vi "System Config_SubVIs-某型振动实验台测试系统.vi"(8 "Error In":errorcluster) -> (0 "Error Out":errorcluster, 1 "Cancle":bool, 3 "Task Info":T1={"Accele Task"=[], "Simulate"=FALSE, "采样率"={"AISampleRate"=10123, "CouplingType"=10000, "Butter"=1000}, "Trig"={"PreTrigCNT"=0, "TriggerMode"=enum."中间触发", "TriggerSource"=enum."软件触发", "ATRTriggerChannel"=enum."通道0", "TriggerDir"=enum."下降沿触发", "TrigLevelVolt"=0.0, "bAvailableTrig"=FALSE}, "clock"={"EN"=FALSE, "clocksource"=enum."内部时钟", "outclocksource"=enum."Trig0"}, "delay(S)"=0.0} {"采样率"."CouplingType" items=["直流耦合", "交流耦合"]})   [LabVIEW 2011]
uses:
  Ctrls/Task Info.ctl
  Ctrls/Sample Information.ctl
  Ctrls/Trig.ctl
  Ctrls/clock.ctl
  Ctrls/task.ctl
  Ctrls/DATA info.ctl
panel:
  in  "取消":bool
  in  "确认":bool
  in  "Tab Control":enum32{"通道设置", "硬件设置"}(tab)
  in  "Scrollbar":i32(c297)
  in  "Accele":T2[](array[typedef])=[{"Enable"=FALSE, "Name"="", "range"=enum."±1V", "SensValue"=0.0, "PhysicalName"="", "off"=0.0, "Sensunits"=""}, {"Enable"=FALSE, "Name"="", "range"=enum."±1V", "SensValue"=0.0, "PhysicalName"="", "off"=0.0, "Sensunits"=""}, {"Enable"=FALSE, "Name"="", "range"=enum."±1V", "SensValue"=0.0, "PhysicalName"="", "off"=0.0, "Sensunits"=""}, {"Enable"=FALSE, "Name"="", "range"=enum."±1V", "SensValue"=0.0, "PhysicalName"="", "off"=0.0, "Sensunits"=""}]
  in  "All":bool caption="选择全部"
  in  "triglevelvolt":dbl caption="触发值(Mpa)"
  in  "数据保存时间(S)":dbl
  in  "Trig.ctlclock":T5
  in  "SampleInfo":T3={"AISampleRate"=10123, "CouplingType"=10000, "Butter"=1000} {"CouplingType" items=["直流耦合", "交流耦合"]; "AISampleRate" format="%#_6f"}
  in  "PreTrigCNT":i32 caption="预触发数"
  in  "TriggerMode":enum16{"中间触发", "后触发", "预触发", "硬件延时触发"}(ring) caption="触发模式"
  in  "TriggerSource":enum16{"软件触发", "DTR信号源", "ATR信号源", "Triger信号触发"}(ring) caption="触发源"
  in  "ATRTriggerChannel":enum16{"通道0", "通道1", "通道2", "通道3"}(ring) caption="触发通道"
  in  "TriggerDir":enum16{"下降沿触发", "上升沿触发", "上下边没均触发"}(ring) caption="触发方向"
  in  "bAvailableTrig":bool caption="触发事件提前有效么？"
  # "增益"
  # "使用"
  # "物理通道"
  # "通道名称"
  # "灵敏度"
  # "偏差"
  # "单位"
  # "采样"
  # "触发"
  # "时钟"
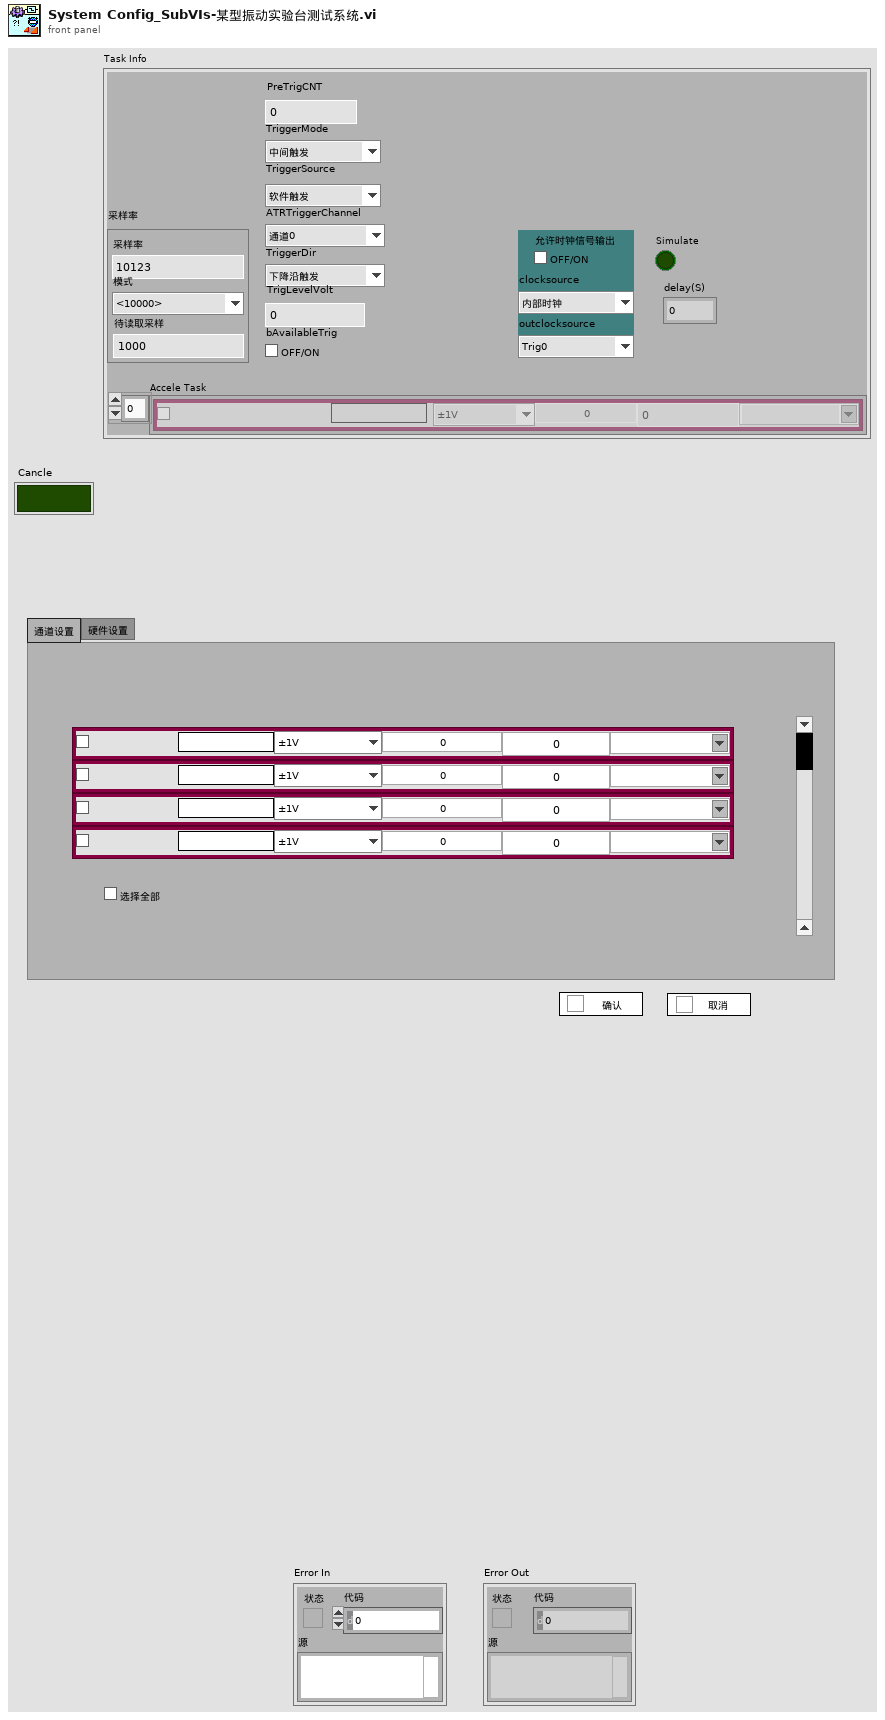
[diagram p1: front panel]
types:
  T1 = typedef "Task Info.ctl" = cluster{"Accele Task":T2[], "Simulate":bool, "采样率":T3, "Trig":T4, "clock":T5, "delay(S)":dbl}
  T2 = typedef "Acceleration Channel Config_Ctrls-某型振动实验台测试系统.ctl" = cluster{"Enable":bool, "Name":string, "range":enum16{"±1V", "±5V"}, "SensValue":dbl, "PhysicalName":string, "off":dbl, "Sensunits":string}
  T3 = typedef "Sample Information.ctl" = cluster{"AISampleRate":i32, "CouplingType":i32, "Butter":i32}
  T4 = typedef "Trig.ctl" = cluster{"PreTrigCNT":i32, "TriggerMode":enum16{"中间触发", "后触发", "预触发", "硬件延时触发"}, "TriggerSource":enum16{"软件触发", "DTR信号源", "ATR信号源", "Triger信号触发"}, "ATRTriggerChannel":enum16{"通道0", "通道1", "通道2", "通道3"}, "TriggerDir":enum16{"下降沿触发", "上升沿触发", "上下边没均触发"}, "TrigLevelVolt":sgl, "bAvailableTrig":bool}
  T5 = typedef "clock.ctl" = cluster{"EN":bool, "clocksource":enum16{"内部时钟", "外部时钟"}, "outclocksource":enum16{"Trig0", "Trig1", "Trig2", "Trig3", "Trig4", "Trig5", "Trig6", "Trig7", "PXI_STAR"}}
  T6 = typedef "Enum Config_Ctrls-某型振动实验台测试系统.ctl" = enum16{"Initialize", "No Action", "Save Config File", "Error Handle", "Exit"}
  T7 = typedef "task.ctl" = cluster{"Task Info":T1, "datain":T8, "times":dbl, "timer":timestamp[], "\nen":bool}
  T8 = typedef "DATA info.ctl" = cluster{"nSegmentCount":i32, "chaneldataSize":i32, "t0 in":timestamp, "nsegmentsize":i32, "chanelcouter":i32}
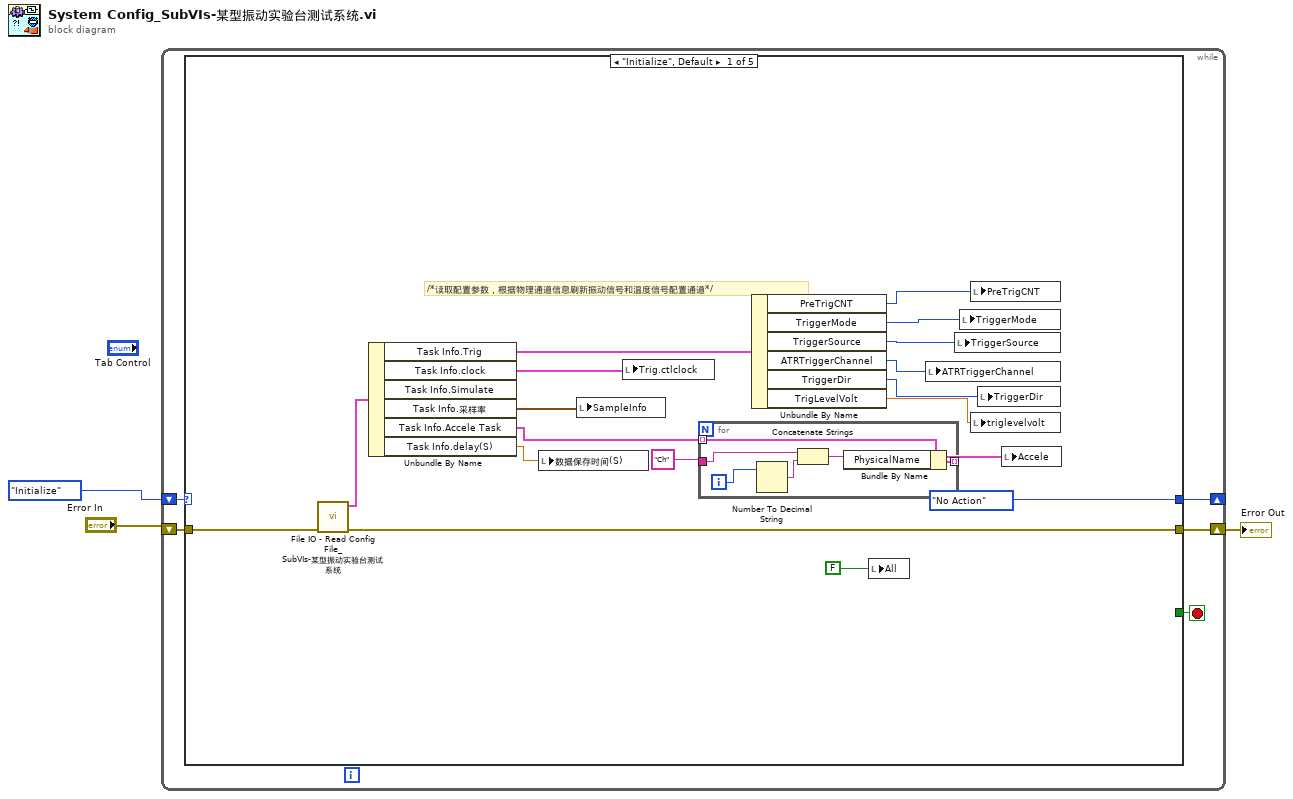
[diagram p0: block diagram]
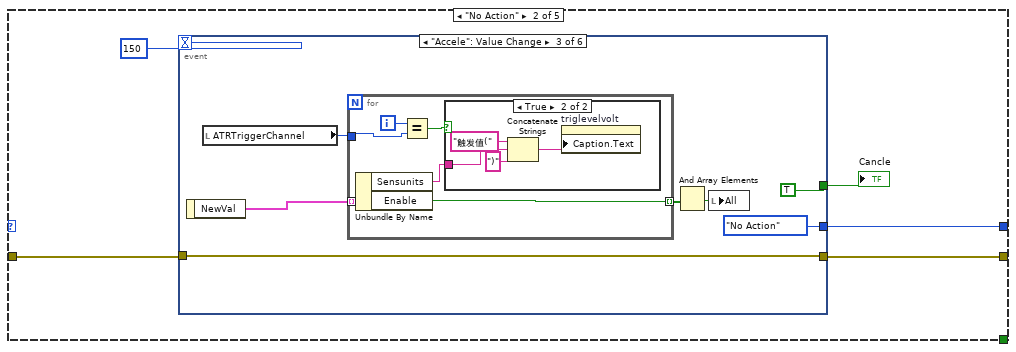
[diagram p2: hidden frame]
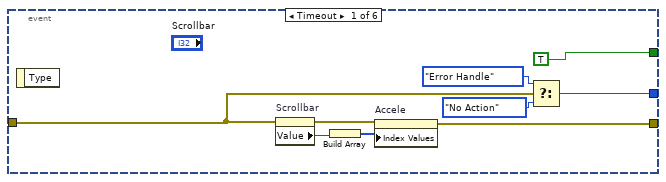
[diagram p3: hidden frame]
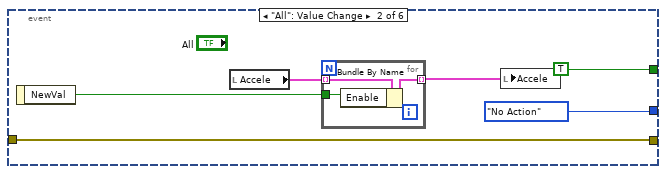
[diagram p4: hidden frame]
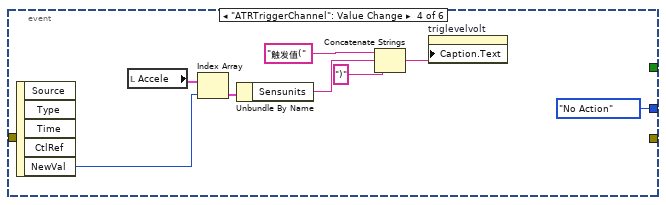
[diagram p6: hidden frame]
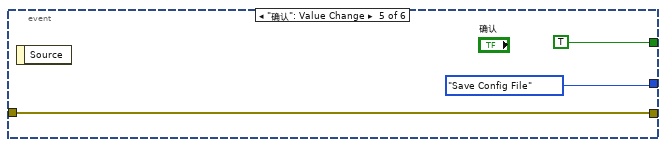
[diagram p7: hidden frame]
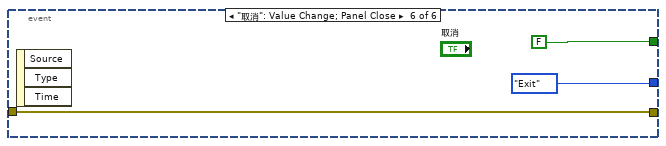
[diagram p8: hidden frame]
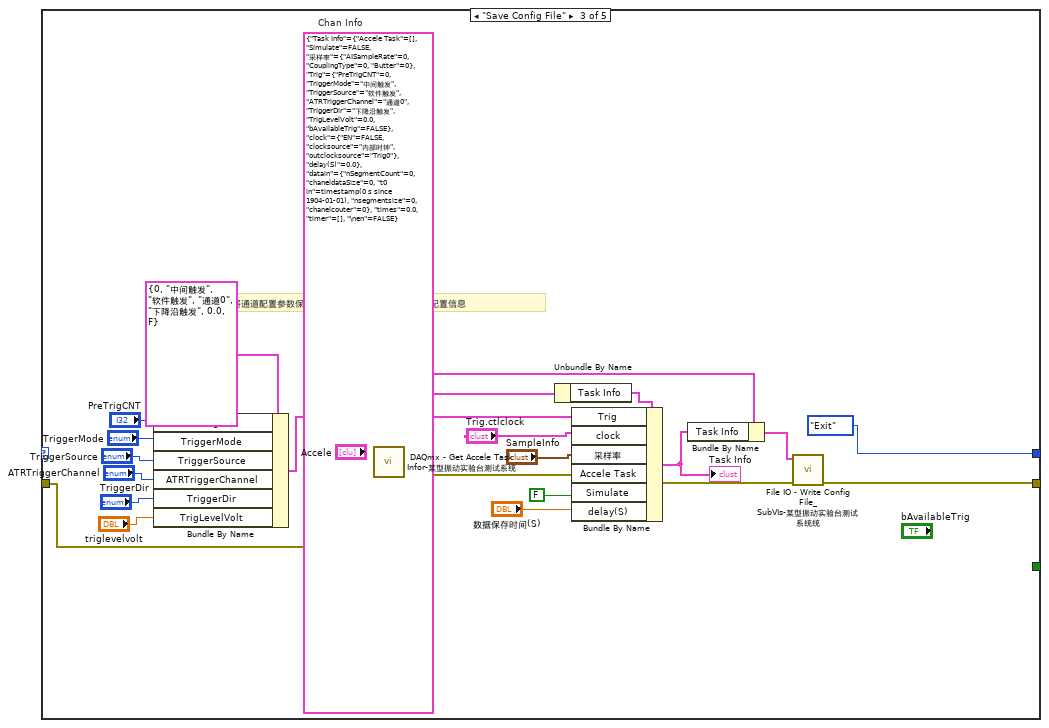
[diagram p9: hidden frame]
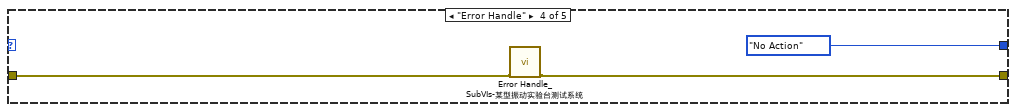
[diagram p10: hidden frame]
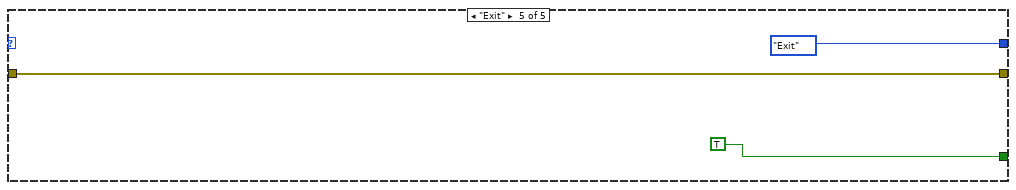
[diagram p11: hidden frame]
diagram:
  n1 = while {
    shift-right: [w6] -> w1
    shift-left: "Error In" -> [w7]
    shift-right: [w5] -> _
    shift-left: Enum_Config_Ctrls-某型振动实验台测试系统."Initialize" ("Enum") -> [w8]
    stop <- w4 stop-if-true
    n2 = case shown="\"Initialize\", Default" w8 {
      tunnel: w7 -> [w23 w36 w106 w110 w113]
      tunnel: [w21 w35 w108 w109 w113] -> w6
      tunnel: [Enum_Config_Ctrls-某型振动实验台测试系统."No Action" ("Enum") w34 Enum_Config_Ctrls-某型振动实验台测试系统."Exit" ("Enum") Enum_Config_Ctrls-某型振动实验台测试系统."No Action" ("Enum") Enum_Config_Ctrls-某型振动实验台测试系统."Exit" ("Enum")] -> w5
      tunnel: [_ _ _ _ TRUE] -> w4
      frame "Initialize", Default {
        # "/*读取配置参数，根据物理通道信息刷新振动信号和温度信号配置通道*/"
        n3 = call "File IO - Read Config File_SubVIs-某型振动实验台测试系统.vi"("Error In"=w23) -> ("Error Out"=w21:errorcluster, "Chan info Output"=w10:T7)  [unwired: 7 out]
        n4 = Unbundle By Name(w10) -> ("Task Info.Trig"=w17:T4, "Task Info.clock"=w19:T5, "Task Info.采样率"=w20:T3, "Task Info.Accele Task"=w26:T2[], "Task Info.delay(S)"=w9:dbl)  [unwired: 1 out]
        n5 = local write "数据保存时间(S)"(w9) -> ()
        n6 = local write "SampleInfo"(w20) -> ()
        n7 = local write "Trig.ctlclock"(w19) -> ()
        n8 = for {
          tunnel: w26 -> [w32] mode=indexing
          tunnel: [w31] -> w22 mode=indexing
          tunnel: "Ch" -> [w29]
          i -> [w30]
          n9 = Number To Decimal String(number=w30) -> (decimal integer string=w28:string)  [unwired: 1 out]
          n10 = Concatenate Strings(w29, w28) -> (w27:string)
          n11 = Bundle By Name(cluster=w32, "PhysicalName"=w27) -> (w31:T2)
        }
        n12 = Unbundle By Name(w17) -> ("PreTrigCNT"=w16:i32, "TriggerMode"=w15:enum16{"中间触发", "后触发", "预触发", "硬件延时触发"}, "TriggerSource"=w13:enum16{"软件触发", "DTR信号源", "ATR信号源", "Triger信号触发"}, "ATRTriggerChannel"=w12:enum16{"通道0", "通道1", "通道2", "通道3"}, "TriggerDir"=w14:enum16{"下降沿触发", "上升沿触发", "上下边没均触发"}, "TrigLevelVolt"=w11:sgl)
        n13 = local write "All"(FALSE ("选择全部")) -> ()
        n14 = local write "ATRTriggerChannel"(w12) -> ()
        n15 = local write "TriggerSource"(w13) -> ()
        n16 = local write "TriggerMode"(w15) -> ()
        n17 = local write "PreTrigCNT"(w16) -> ()
        n18 = local write "triglevelvolt"(w11) -> ()
        n19 = local write "TriggerDir"(w14) -> ()
        n20 = local write "Accele"(w22) -> ()
      }
      frame "No Action" {
        n21 = event shown="[2] \"Accele\": Value Change" {
          selector: _ -> [_ _ _ _ _ _]
          dyn-events: _ -> [_ _ _ _ _ _]
          timeout: 150 -> [_ _ _ _ _ _]
          tunnel: w36 -> [w43 w50 w58 _ w82 w86]
          tunnel: [w44 w50 w58 _ w82 w86] -> w35
          tunnel: [w40 Enum_Config_Ctrls-某型振动实验台测试系统."No Action" ("Enum") Enum_Config_Ctrls-某型振动实验台测试系统."No Action" ("Enum") Enum_Config_Ctrls-某型振动实验台测试系统."No Action" ("Enum") Enum_Config_Ctrls-某型振动实验台测试系统."Save Config File" ("Enum") Enum_Config_Ctrls-某型振动实验台测试系统."Exit" ("Enum")] -> w34
          tunnel: [TRUE TRUE TRUE _ TRUE FALSE] -> w33
          event Timeout {
            n22 = event-data() -> ()  [unwired: 2 out]
            n23 = property on="Scrollbar" class="Scroll (strict)"(error in=w43) -> (error out=w45:errorcluster, "Value"=w39:i32)  [unwired: 1 in, 1 out]
            n24 = Build Array(w39) -> (w46:i32[])
            n25 = property on="Accele" class="Arr (strict)"(error in=w45, "Index Values"=w46) -> (error out=w44:errorcluster)  [unwired: 1 in, 1 out]
            n26 = Select(t=Enum_Config_Ctrls-某型振动实验台测试系统."Error Handle" ("Enum"), s=w43, f=Enum_Config_Ctrls-某型振动实验台测试系统."No Action" ("Enum")) -> (s? t:f=w40:T6)
          }
          event "All": Value Change {
            n27 = event-data() -> ("NewVal"=w52:bool)  [unwired: 1 out]
            n28 = local read "Accele"() -> (w49:T2[])
            n29 = for {
              tunnel: w52 -> [w54]
              tunnel: w49 -> [w55] mode=indexing
              tunnel: [w53] -> w48 mode=indexing
              n30 = Bundle By Name(cluster=w55, "Enable"=w54) -> (w53:T2)
            }
            n31 = local write "Accele"(w48) -> ()
          }
          event "Accele": Value Change {
            n32 = event-data() -> ("NewVal"=w62:T2[])  [unwired: 1 out]
            n33 = local read "ATRTriggerChannel"() -> (w56:enum16{"通道0", "通道1", "通道2", "通道3"})
            n34 = for {
              tunnel: w62 -> [w68] mode=indexing
              tunnel: [w67] -> w61 mode=indexing
              tunnel: w56 -> [w65]
              i -> [w66]
              n35 = Unbundle By Name(w68) -> ("Sensunits"=w63:string, "Enable"=w67:bool)
              n36 = Equal?(x=w66, y=w65) -> (x = y?=w64:bool)
              n37 = case shown="True" w64 {
                tunnel: w63 -> [_ w71]
                frame False {
                }
                frame True {
                  n38 = Concatenate Strings("触发值(" ("字符串"), w71, ")" ("字符串")) -> (w72:string)
                  n39 = property on="triglevelvolt" class="DigNum (strict)"("Caption.Text"=w72) -> ()  [unwired: 2 in, 2 out]
                }
              }
            }
            n40 = And Array Elements(Boolean array=w61) -> (logical AND=w60:bool)
            n41 = local write "All"(w60) -> ()
          }
          event "ATRTriggerChannel": Value Change {
            n42 = event-data() -> ("NewVal"=w75:enum16{"通道0", "通道1", "通道2", "通道3"})  [unwired: 5 out]
            n43 = local read "Accele"() -> (w76:T2[])
            n44 = Index Array(array=w76, index=w75) -> (element=w74:T2)
            n45 = Unbundle By Name(w74) -> ("Sensunits"=w73:string)
            n46 = Concatenate Strings("触发值(" ("字符串"), w73, ")" ("字符串")) -> (w79:string)
            n47 = property on="triglevelvolt" class="DigNum (strict)"("Caption.Text"=w79) -> ()  [unwired: 2 in, 2 out]
          }
          event "确认": Value Change {
            n48 = event-data() -> ()  [unwired: 2 out]
          }
          event "取消": Value Change; Panel Close {
            n49 = event-data() -> ()  [unwired: 4 out]
          }
        }
        "Cancle" <- w33
      }
      frame "Save Config File" {
        w87 = T7 {"Task Info"={"Accele Task"=[], "Simulate"=FALSE, "采样率"={"AISampleRate"=0, "CouplingType"=0, "Butter"=0}, "Trig"={"PreTrigCNT"=0, "TriggerMode"=enum."中间触发", "TriggerSource"=enum."软件触发", "ATRTriggerChannel"=enum."通道0", "TriggerDir"=enum."下降沿触发", "TrigLevelVolt"=0.0, "bAvailableTrig"=FALSE}, "clock"={"EN"=FALSE, "clocksource"=enum."内部时钟", "outclocksource"=enum."Trig0"}, "delay(S)"=0.0}, "datain"={"nSegmentCount"=0, "chaneldataSize"=0, "t0 in"=timestamp(0 s since 1904-01-01), "nsegmentsize"=0, "chanelcouter"=0}, "times"=0.0, "timer"=[], "\nen"=FALSE}  # Chan Info
        # "将通道配置参数保存至配置文件，并输出当前任务配置信息"
        n50 = Bundle By Name(cluster=T4 {"PreTrigCNT"=0, "TriggerMode"=enum."中间触发", "TriggerSource"=enum."软件触发", "ATRTriggerChannel"=enum."通道0", "TriggerDir"=enum."下降沿触发", "TrigLevelVolt"=0.0, "bAvailableTrig"=FALSE} ("Trig"), "PreTrigCNT"="PreTrigCNT", "TriggerMode"="TriggerMode", "TriggerSource"="TriggerSource", "ATRTriggerChannel"="ATRTriggerChannel", "TriggerDir"="TriggerDir", "TrigLevelVolt"="triglevelvolt") -> (w89:T4)
        n51 = call "DAQmx - Get Accele Task Infor-某型振动实验台测试系统.vi"("error in (no error)"=w106, "Accele"="Accele") -> ("error out"=w105:errorcluster, "PXI-4498 Task"=w103:T2[])  [unwired: 8 out]
        n52 = Unbundle By Name(w87) -> ("Task Info"=w100:T1)
        n53 = Bundle By Name(cluster=w100, "Trig"=w89, "clock"="Trig.ctlclock", "采样率"="SampleInfo", "Accele Task"=w103, "Simulate"=FALSE ("Simulate？"), "delay(S)"="数据保存时间(S)") -> (w98:T1)
        "Task Info" <- w98
        n54 = Bundle By Name(cluster=w87, "Task Info"=w98) -> (w99:T7)
        n55 = call "File IO - Write Config File_SubVIs-某型振动实验台测试系统统.vi"("Error In"=w105, "Chan Info"=w99) -> ("Error Out"=w108:errorcluster)  [unwired: 1 in, 8 out]
      }
      frame "Error Handle" {
        n56 = call "Error Handle_SubVIs-某型振动实验台测试系统.vi"("error in"=w110) -> ("error out"=w109:errorcluster)  [unwired: 10 out]
      }
      frame "Exit" {
      }
    }
  }
  "Error Out" <- w1
